vi "NetComm_getJoystickPOVs.vi"(8 "error in (no error)":errorcluster, 11 "Joystick Number":i32) -> (0 "error out":errorcluster, 2 "POVs":i16[](array[numeric]))   [LabVIEW 2017]
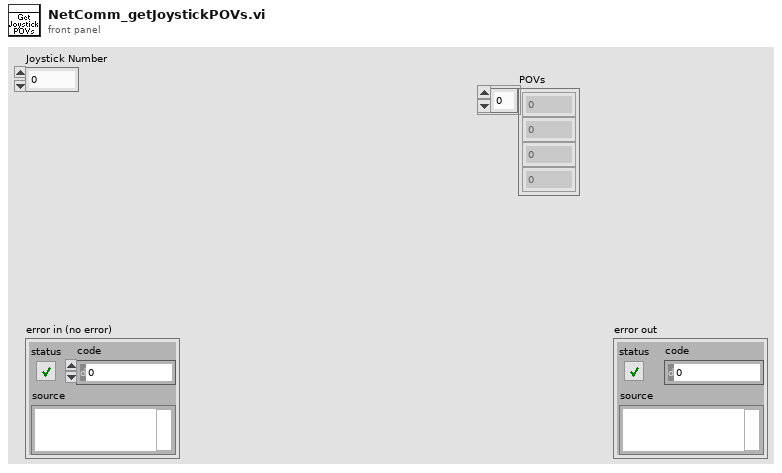
[diagram p1: front panel]
types:
  T1 = enum16{"big-endian, network order", "native, host order", "little-endian"}
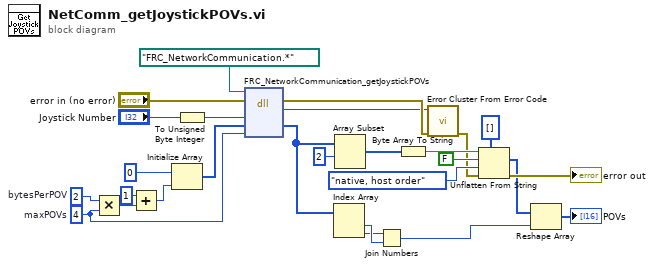
[diagram p0: block diagram]
diagram:
  w25 = u8 2  # bytesPerPOV
  w4 = u8 4  # maxPOVs
  n1 = Multiply(x=w25, y=w4) -> (x*y=w24:u8)
  n2 = Add(x=u8 1, y=w24) -> (x+y=w22:u8)
  n3 = Initialize Array(u8 0, w22) -> (w5:u8[])
  n4 = To Unsigned Byte Integer(number="Joystick Number") -> (unsigned 8bit integer=w6:u8)
  n5 = dll-call lib="?" fn="FRC_NetworkCommunication_getJoystickPOVs"(path in=path "FRC_NetworkCommunication.*", error in="error in (no error)", "joystickNum"=w6, "povs"=w5, "maxPOVs"=w4) -> (error out=w9:errorcluster, "return type"=w8:i32, "povs"=w7:u8[])  [unwired: 3 in, 1 out]
  n6 = Index Array(array=w7) -> (element #1=w3:u8, element #2=w2:u8)  [unwired: 2 in]
  n7 = Array Subset(array=w7, index=2) -> (w15:u8[])  [unwired: 1 in]
  n8 = Join Numbers(hi=w2, lo=w3) -> ((hi.lo)=w1:u16)
  n9 = Byte Array To String(unsigned byte array=w15) -> (string=w20:string)
  n10 = call <vilib>:"Error Cluster From Error Code.vi"("error in (no error)"=w9, "error code (0)"=w8) -> ("error out"=w17:errorcluster)  [unwired: 7 in]
  n11 = Unflatten From String(type=i16[] [], binary string=w20, data includes array or string size? (T)=FALSE, byte order (0:big-endian, network order)=T1."native, host order", error in (no error)=w17) -> (value=w13:i16[], error out=→"error out":errorcluster)  [unwired: 1 out]
  n12 = Reshape Array(w13, w1) -> (→"POVs":i16[])
